vi "GeoData.vi"() -> ()   [LabVIEW 2017] (continued)
GA\tMadison County\tH1\n30530\t13195\tCommerce\tGA\tMadison County\tH1\n30629\t13195\tComer\tGA\tMadison County\tH1\n30624\t13195\tBowman\tGA\tMadison County\tH1\n30601\t13195\tAthens\tGA\tMadison County\tH1\n30646\t13195\tHull\tGA\tMadison County\tH1\n30662\t13195\tRoyston\tGA\tMadison County\tH1\n30647\t13195\tIla\tGA\tMadison County\tH1\n31801\t13197\tBox springs\tGA\tMarion County\tH1\n31805\t13197\tCusseta\tGA\tMarion County\tH1\n31803\t13197\tBuena vista\tGA\tMarion County\tH1\n31058\t13197\tMauk\tGA\tMarion County\tH1\n31824\t13197\tPreston\tGA\tMarion County\tH1\n30241\t13199\tLagrange\tGA\tMeriwether County\tH1\n30251\t13199\tLuthersville\tGA\tMeriwether County\tH1\n30230\t13199\tHogansville\tGA\tMeriwether County\tH1\n30293\t13199\tWoodbury\tGA\tMeriwether County\tH1\n31822\t13199\tPine mountain\tGA\tMeriwether County\tH1\n31816\t13199\tManchester\tGA\tMeriwether County\tH1\n30220\t13199\tGrantville\tGA\tMeriwether County\tH1\n30276\t13199\tSenoia\tGA\tMeriwether County\tH1\n30259\t13199\tMoreland\tGA\tMeriwether County\tH1\n30218\t13199\tGay\tGA\tMeriwether County\tH1\n30222\t13199\tGreenville\tGA\tMeriwether County\tH1\n31830\t13199\tWarm springs\tGA\tMeriwether County\tH1\n39841\t13201\tDamascus\tGA\tMiller County\tH1\n39859\t13201\tIron city\tGA\tMiller County\tH1\n39823\t13201\tBlakely\tGA\tMiller County\tH1\n39845\t13201\tDonalsonville\tGA\tMiller County\tH1\n39837\t13201\tColquitt\tGA\tMiller County\tH1\n31744\t13205\tDoerun\tGA\tMitchell County\tH1\n31779\t13205\tPelham\tGA\tMitchell County\tH1\n31784\t13205\tSale city\tGA\tMitchell County\tH1\n31765\t13205\tMeigs\tGA\tMitchell County\tH1\n31716\t13205\tBaconton\tGA\tMitchell County\tH1\n31705\t13205\tAlbany\tGA\tMitchell County\tH1\n31730\t13205\tCamilla\tGA\tMitchell County\tH1\n31016\t13207\tCulloden\tGA\tMonroe County\tH1\n31097\t13207\tYatesville\tGA\tMonroe County\tH1\n30204\t13207\tBarnesville\tGA\tMonroe County\tH1\n31220\t13207\tMacon\tGA\tMonroe County\tH1\n31029\t13207\tForsyth\tGA\tMonroe County\tH1\n31046\t13207\tJuliette\tGA\tMonroe County\tH1\n31066\t13207\tMusella\tGA\tMonroe County\tH1\n31086\t13207\tSmarr\tGA\tMonroe County\tH1\n30233\t13207\tJackson\tGA\tMonroe County\tH1\n31210\t13207\tMacon\tGA\tMonroe County\tH1\n31004\t13207\tBolingbroke\tGA\tMonroe County\tH1\n30457\t13209\tSoperton\tGA\tMontgomery County\tH1\n30445\t13209\tMount vernon\tGA\tMontgomery County\tH1\n30470\t13209\tTarrytown\tGA\tMontgomery County\tH1\n30410\t13209\tAiley\tGA\tMontgomery County\tH1\n30473\t13209\tUvalda\tGA\tMontgomery County\tH1\n30412\t13209\tAlston\tGA\tMontgomery County\tH1\n30474\t13209\tVidalia\tGA\tMontgomery County\tH1\n30625\t13211\tBuckhead\tGA\tMorgan County\tH1\n30623\t13211\tBostwick\tGA\tMorgan County\tH1\n30055\t13211\tMansfield\tGA\tMorgan County\tH1\n30650\t13211\tMadison\tGA\tMorgan County\tH1\n30025\t13211\tSocial circle\tGA\tMorgan County\tH1\n30663\t13211\tRutledge\tGA\tMorgan County\tH1\n30056\t13211\tNewborn\tGA\tMorgan County\tH1\n30621\t13211\tBishop\tGA\tMorgan County\tH1\n30641\t13211\tGood hope\tGA\tMorgan County\tH1\n30711\t13213\tCrandall\tGA\tMurray County\tH1\n30705\t13213\tChatsworth\tGA\tMurray County\tH1\n30751\t13213\tTennga\tGA\tMurray County\tH1\n30540\t13213\tEllijay\tGA\tMurray County\tH1\n30708\t13213\tCisco\tGA\tMurray County\tH1\n30735\t13213\tResaca\tGA\tMurray County\tH1\n30721\t13213\tDalton\tGA\tMurray County\tH1\n30724\t13213\tEton\tGA\tMurray County\tH1\n31801\t13215\tBox springs\tGA\tMuscogee County\tH6\n31905\t13215\tFort benning\tGA\tMuscogee County\tH6\n31908\t13215\tColumbus\tGA\tMuscogee County\tH6\n31914\t13215\tColumbus\tGA\tMuscogee County\tH6\n31999\t13215\tColumbus\tGA\tMuscogee County\tH6\n31808\t13215\tFortson\tGA\tMuscogee County\tH6\n31804\t13215\tCataula\tGA\tMuscogee County\tH6\n31901\t13215\tColumbus\tGA\tMuscogee County\tH6\n31917\t13215\tColumbus\tGA\tMuscogee County\tH6\n31998\t13215\tColumbus\tGA\tMuscogee County\tH6\n31903\t13215\tColumbus\tGA\tMuscogee County\tH6\n31904\t13215\tColumbus\tGA\tMuscogee County\tH6\n31909\t13215\tColumbus\tGA\tMuscogee County\tH6\n31902\t13215\tColumbus\tGA\tMuscogee County\tH6\n31820\t13215\tMidland\tGA\tMuscogee County\tH6\n31906\t13215\tColumbus\tGA\tMuscogee County\tH6\n31907\t13215\tColumbus\tGA\tMuscogee County\tH6\n31829\t13215\tUpatoi\tGA\tMuscogee County\tH6\n30014\t13217\tCovington\tGA\tNewton County\tH1\n30016\t13217\tCovington\tGA\tNewton County\tH1\n30013\t13217\tConyers\tGA\tNewton County\tH1\n30055\t13217\tMansfield\tGA\tNewton County\tH1\n31064\t13217\tMonticello\tGA\tNewton County\tH1\n30015\t13217\tCovington\tGA\tNewton County\tH1\n30070\t13217\tPorterdale\tGA\tNewton County\tH1\n30025\t13217\tSocial circle\tGA\tNewton County\tH1\n30052\t13217\tLoganville\tGA\tNewton County\tH1\n30094\t13217\tConyers\tGA\tNewton County\tH1\n30054\t13217\tOxford\tGA\tNewton County\tH1\n30056\t13217\tNewborn\tGA\tNewton County\tH1\n30233\t13217\tJackson\tGA\tNewton County\tH1\n30638\t13219\tFarmington\tGA\tOconee County\tH1\n30677\t13219\tWatkinsville\tGA\tOconee County\tH1\n30605\t13219\tAthens\tGA\tOconee County\tH1\n30606\t13219\tAthens\tGA\tOconee County\tH1\n30622\t13219\tBogart\tGA\tOconee County\tH1\n30619\t13219\tArnoldsville\tGA\tOconee County\tH1\n30645\t13219\tHigh shoals\tGA\tOconee County\tH1\n30680\t13219\tWinder\tGA\tOconee County\tH1\n30666\t13219\tStatham\tGA\tOconee County\tH1\n30621\t13219\tBishop\tGA\tOconee County\tH1\n30630\t13221\tCrawford\tGA\tOglethorpe County\tH1\n30627\t13221\tCarlton\tGA\tOglethorpe County\tH1\n30628\t13221\tColbert\tGA\tOglethorpe County\tH1\n30648\t13221\tLexington\tGA\tOglethorpe County\tH1\n30667\t13221\tStephens\tGA\tOglethorpe County\tH1\n30683\t13221\tWinterville\tGA\tOglethorpe County\tH1\n30619\t13221\tArnoldsville\tGA\tOglethorpe County\tH1\n30629\t13221\tComer\tGA\tOglethorpe County\tH1\n30660\t13221\tRayle\tGA\tOglethorpe County\tH1\n30669\t13221\tUnion point\tGA\tOglethorpe County\tH1\n30134\t13223\tDouglasville\tGA\tPaulding County\tH1\n30132\t13223\tDallas\tGA\tPaulding County\tH1\n30157\t13223\tDallas\tGA\tPaulding County\tH1\n30179\t13223\tTemple\tGA\tPaulding County\tH1\n30127\t13223\tPowder springs\tGA\tPaulding County\tH1\n30178\t13223\tTaylorsville\tGA\tPaulding County\tH1\n30101\t13223\tAcworth\tGA\tPaulding County\tH1\n30180\t13223\tVilla rica\tGA\tPaulding County\tH1\n30120\t13223\tCartersville\tGA\tPaulding County\tH1\n30141\t13223\tHiram\tGA\tPaulding County\tH1\n30153\t13223\tRockmart\tGA\tPaulding County\tH1\n31076\t13225\tReynolds\tGA\tPeach County\tH1\n31069\t13225\tPerry\tGA\tPeach County\tH1\n31008\t13225\tByron\tGA\tPeach County\tH1\n31030\t13225\tFort valley\tGA\tPeach County\tH1\n30534\t13227\tDawsonville\tGA\tPickens County\tH1\n30107\t13227\tBall ground\tGA\tPickens County\tH1\n30536\t13227\tEllijay\tGA\tPickens County\tH1\n30139\t13227\tFairmount\tGA\tPickens County\tH1\n30177\t13227\tTate\tGA\tPickens County\tH1\n30540\t13227\tEllijay\tGA\tPickens County\tH1\n30183\t13227\tWaleska\tGA\tPickens County\tH1\n30734\t13227\tRanger\tGA\tPickens County\tH1\n30143\t13227\tJasper\tGA\tPickens County\tH1\n30148\t13227\tMarble hill\tGA\tPickens County\tH1\n30175\t13227\tTalking rock\tGA\tPickens County\tH1\n31551\t13229\tMershon\tGA\tPierce County\tH1\n31557\t13229\tPatterson\tGA\tPierce County\tH1\n31518\t13229\tBristol\tGA\tPierce County\tH1\n31556\t13229\tOfferman\tGA\tPierce County\tH1\n31516\t13229\tBlackshear\tGA\tPierce County\tH1\n31503\t13229\tWaycross\tGA\tPierce County\tH1\n31510\t13229\tAlma\tGA\tPierce County\tH1\n30206\t13231\tConcord\tGA\tPike County\tH1\n30295\t13231\tZebulon\tGA\tPike County\tH1\n30224\t13231\tGriffin\tGA\tPike County\tH1\n30258\t13231\tMolena\tGA\tPike County\tH1\n30292\t13231\tWilliamson\tGA\tPike County\tH1\n30257\t13231\tMilner\tGA\tPike County\tH1\n30285\t13231\tThe rock\tGA\tPike County\tH1\n30256\t13231\tMeansville\tGA\tPike County\tH1\n30124\t13233\tCave spring\tGA\tPolk County\tH1\n30147\t13233\tLindale\tGA\tPolk County\tH1\n30138\t13233\tEsom hill\tGA\tPolk County\tH1\n30178\t13233\tTaylorsville\tGA\tPolk County\tH1\n30125\t13233\tCedartown\tGA\tPolk County\tH1\n30104\t13233\tAragon\tGA\tPolk County\tH1\n30173\t13233\tSilver creek\tGA\tPolk County\tH1\n30113\t13233\tBuchanan\tGA\tPolk County\tH1\n30153\t13233\tRockmart\tGA\tPolk County\tH1\n31036\t13235\tHawkinsville\tGA\tPulaski County\tH1\n31071\t13235\tPineview\tGA\tPulaski County\tH1\n31014\t13235\tCochran\tGA\tPulaski County\tH1\n31091\t13235\tUnadilla\tGA\tPulaski County\tH1\n31023\t13235\tEastman\tGA\tPulaski County\tH1\n30625\t13237\tBuckhead\tGA\tPutnam County\tH1\n31026\t13237\tEatonton\tGA\tPutnam County\tH1\n31024\t13237\tEatonton\tGA\tPutnam County\tH1\n30650\t13237\tMadison\tGA\tPutnam County\tH1\n31061\t13237\tMilledgeville\tGA\tPutnam County\tH1\n39854\t13239\tGeorgetown\tGA\tQuitman County\tH1\n39867\t13239\tMorris\tGA\tQuitman County\tH1\n30568\t13241\tRabun gap\tGA\tRabun County\tH1\n30523\t13241\tClarkesville\tGA\tRabun County\tH1\n30537\t13241\tDillard\tGA\tRabun County\tH1\n30562\t13241\tMountain city\tGA\tRabun County\tH1\n30576\t13241\tTiger\tGA\tRabun County\tH1\n30581\t13241\tWiley\tGA\tRabun County\tH1\n30573\t13241\tTallulah falls\tGA\tRabun County\tH1\n30525\t13241\tClayton\tGA\tRabun County\tH1\n30552\t13241\tLakemont\tGA\tRabun County\tH1\n39840\t13243\tCuthbert\tGA\tRandolph County\tH1\n39866\t13243\tMorgan\tGA\tRandolph County\tH1\n39867\t13243\tMorris\tGA\tRandolph County\tH1\n39846\t13243\tEdison\tGA\tRandolph County\tH1\n39886\t13243\tShellman\tGA\tRandolph County\tH1\n39836\t13243\tColeman\tGA\tRandolph County\tH1\n39851\t13243\tFort gaines\tGA\tRandolph County\tH1\n30912\t13245\tAugusta\tGA\tRichmond County\tH6\n30901\t13245\tAugusta\tGA\tRichmond County\tH6\n30909\t13245\tAugusta\tGA\tRichmond County\tH6\n30815\t13245\tHephzibah\tGA\tRichmond County\tH6\n30906\t13245\tAugusta\tGA\tRichmond County\tH6\n30905\t13245\tAugusta\tGA\tRichmond County\tH6\n30812\t13245\tGracewood\tGA\tRichmond County\tH6\n30805\t13245\tBlythe\tGA\tRichmond County\tH6\n30904\t13245\tAugusta\tGA\tRichmond County\tH6\n30907\t13245\tAugusta\tGA\tRichmond County\tH6\n30903\t13245\tAugusta\tGA\tRichmond County\tH6\n30916\t13245\tAugusta\tGA\tRichmond County\tH6\n30919\t13245\tAugusta\tGA\tRichmond County\tH6\n30914\t13245\tAugusta\tGA\tRichmond County\tH6\n30813\t13245\tGrovetown\tGA\tRichmond County\tH6\n30016\t13247\tCovington\tGA\tRockdale County\tH1\n30039\t13247\tSnellville\tGA\tRockdale County\tH1\n30013\t13247\tConyers\tGA\tRockdale County\tH1\n30012\t13247\tConyers\tGA\tRockdale County\tH1\n30294\t13247\tEllenwood\tGA\tRockdale County\tH1\n30058\t13247\tLithonia\tGA\tRockdale County\tH1\n30052\t13247\tLoganville\tGA\tRockdale County\tH1\n30094\t13247\tConyers\tGA\tRockdale County\tH1\n30252\t13247\tMcdonough\tGA\tRockdale County\tH1\n30281\t13247\tStockbridge\tGA\tRockdale County\tH1\n31711\t13249\tAndersonville\tGA\tSchley County\tH1\n31806\t13249\tEllaville\tGA\tSchley County\tH1\n31081\t13249\tRupert\tGA\tSchley County\tH1\n31068\t13249\tOglethorpe\tGA\tSchley County\tH1\n31719\t13249\tAmericus\tGA\tSchley County\tH1\n31803\t13249\tBuena vista\tGA\tSchley County\tH1\n31058\t13249\tMauk\tGA\tSchley County\tH1\n30424\t13251\tDover\tGA\tScreven County\tH1\n30426\t13251\tGirard\tGA\tScreven County\tH1\n30442\t13251\tMillen\tGA\tScreven County\tH1\n30467\t13251\tSylvania\tGA\tScreven County\tH1\n30455\t13251\tRocky ford\tGA\tScreven County\tH1\n30446\t13251\tNewington\tGA\tScreven County\tH1\n30449\t13251\tOliver\tGA\tScreven County\tH1\n39825\t13253\tBrinson\tGA\tSeminole County\tH1\n39859\t13253\tIron city\tGA\tSeminole County\tH1\n39845\t13253\tDonalsonville\tGA\tSeminole County\tH1\n39861\t13253\tJakin\tGA\tSeminole County\tH1\n30223\t13255\tGriffin\tGA\tSpalding County\tH1\n30266\t13255\tOrchard hill\tGA\tSpalding County\tH1\n30284\t13255\tSunny side\tGA\tSpalding County\tH1\n30224\t13255\tGriffin\tGA\tSpalding County\tH1\n30212\t13255\tExperiment\tGA\tSpalding County\tH1\n30228\t13255\tHampton\tGA\tSpalding County\tH1\n30292\t13255\tWilliamson\tGA\tSpalding County\tH1\n30205\t13255\tBrooks\tGA\tSpalding County\tH1\n30248\t13255\tLocust grove\tGA\tSpalding County\tH1\n30598\t13257\tToccoa falls\tGA\tStephens County\tH1\n30557\t13257\tMartin\tGA\tStephens County\tH1\n30538\t13257\tEastanollee\tGA\tStephens County\tH1\n30577\t13257\tToccoa\tGA\tStephens County\tH1\n39854\t13259\tGeorgetown\tGA\tStewart County\tH1\n31825\t13259\tRichland\tGA\tStewart County\tH1\n31805\t13259\tCusseta\tGA\tStewart County\tH1\n39867\t13259\tMorris\tGA\tStewart County\tH1\n31815\t13259\tLumpkin\tGA\tStewart County\tH1\n31821\t13259\tOmaha\tGA\tStewart County\tH1\n31711\t13261\tAndersonville\tGA\tSumter County\tH1\n31806\t13261\tEllaville\tGA\tSumter County\tH1\n31787\t13261\tSmithville\tGA\tSumter County\tH1\n31735\t13261\tCobb\tGA\tSumter County\tH1\n31719\t13261\tAmericus\tGA\tSumter County\tH1\n31709\t13261\tAmericus\tGA\tSumter County\tH1\n31780\t13261\tPlains\tGA\tSumter County\tH1\n31743\t13261\tDe soto\tGA\tSumter County\tH1\n31764\t13261\tLeslie\tGA\tSumter County\tH1\n31801\t13263\tBox springs\tGA\tTalbot County\tH1\n31827\t13263\tTalbotton\tGA\tTalbot County\tH1\n31816\t13263\tManchester\tGA\tTalbot County\tH1\n31826\t13263\tShiloh\tGA\tTalbot County\tH1\n31836\t13263\tWoodland\tGA\tTalbot County\tH1\n31812\t13263\tJunction city\tGA\tTalbot County\tH1\n31810\t13263\tGeneva\tGA\tTalbot County\tH1\n31831\t13263\tWaverly hall\tGA\tTalbot County\tH1\n30673\t13265\tWashington\tGA\tTaliaferro County\tH1\n30678\t13265\tWhite plains\tGA\tTaliaferro County\tH1\n30664\t13265\tSharon\tGA\tTaliaferro County\tH1\n30631\t13265\tCrawfordville\tGA\tTaliaferro County\tH1\n30660\t13265\tRayle\tGA\tTaliaferro County\tH1\n30669\t13265\tUnion point\tGA\tTaliaferro County\tH1\n30420\t13267\tCobbtown\tGA\tTattnall County\tH1\n30421\t13267\tCollins\tGA\tTattnall County\tH1\n30436\t13267\tLyons\tGA\tTattnall County\tH1\n30453\t13267\tReidsville\tGA\tTattnall County\tH1\n30499\t13267\tReidsville\tGA\tTattnall County\tH1\n30417\t13267\tClaxton\tGA\tTattnall County\tH1\n30427\t13267\tGlennville\tGA\tTattnall County\tH1\n30438\t13267\tManassas\tGA\tTattnall County\tH1\n31076\t13269\tReynolds\tGA\tTaylor County\tH1\n31081\t13269\tRupert\tGA\tTaylor County\tH1\n31068\t13269\tOglethorpe\tGA\tTaylor County\tH1\n31041\t13269\tIdeal\tGA\tTaylor County\tH1\n31006\t13269\tButler\tGA\tTaylor County\tH1\n31058\t13269\tMauk\tGA\tTaylor County\tH1\n31812\t13269\tJunction city\tGA\tTaylor County\tH1\n31039\t13269\tHoward\tGA\tTaylor County\tH1\n31037\t13271\tMc rae helena\tGA\tTelfair County\tH1\n31055\t13271\tMc rae helena\tGA\tTelfair County\tH1\n31060\t13271\tMilan\tGA\tTelfair County\tH1\n31549\t13271\tLumber city\tGA\tTelfair County\tH1\n31083\t13271\tScotland\tGA\tTelfair County\tH1\n31077\t13271\tRhine\tGA\tTelfair County\tH1\n31544\t13271\tJacksonville\tGA\tTelfair County\tH1\n31721\t13273\tAlbany\tGA\tTerrell County\tH1\n39842\t13273\tDawson\tGA\tTerrell County\tH1\n39862\t13273\tLeary\tGA\tTerrell County\tH1\n39826\t13273\tBronwood\tGA\tTerrell County\tH1\n39886\t13273\tShellman\tGA\tTerrell County\tH1\n39877\t13273\tParrott\tGA\tTerrell County\tH1\n39885\t13273\tSasser\tGA\tTerrell County\tH1\n31738\t13275\tCoolidge\tGA\tThomas County\tH1\n31720\t13275\tBarwick\tGA\tThomas County\tH1\n31779\t13275\tPelham\tGA\tThomas County\tH1\n31778\t13275\tPavo\tGA\tThomas County\tH1\n31773\t13275\tOchlocknee\tGA\tThomas County\tH1\n31792\t13275\tThomasville\tGA\tThomas County\tH1\n31757\t13275\tThomasville\tGA\tThomas County\tH1\n31765\t13275\tMeigs\tGA\tThomas County\tH1\n39828\t13275\tCairo\tGA\tThomas County\tH1\n31799\t13275\tThomasville\tGA\tThomas County\tH1\n31626\t13275\tBoston\tGA\tThomas County\tH1\n31733\t13277\tChula\tGA\tTift County\tH1\n31775\t13277\tOmega\tGA\tTift County\tH1\n31793\t13277\tTifton\tGA\tTift County\tH1\n31714\t13277\tAshburn\tGA\tTift County\tH1\n31790\t13277\tSycamore\tGA\tTift County\tH1\n31637\t13277\tLenox\tGA\tTift County\tH1\n31795\t13277\tTy ty\tGA\tTift County\tH1\n31727\t13277\tBrookfield\tGA\tTift County\tH1\n31749\t13277\tEnigma\tGA\tTift County\tH1\n31794\t13277\tTifton\tGA\tTift County\tH1\n30436\t13279\tLyons\tGA\tToombs County\tH1\n30453\t13279\tReidsville\tGA\tToombs County\tH1\n30473\t13279\tUvalda\tGA\tToombs County\tH1\n30474\t13279\tVidalia\tGA\tToombs County\tH1\n30582\t13281\tYoung harris\tGA\tTowns County\tH1\n30525\t13281\tClayton\tGA\tTowns County\tH1\n30546\t13281\tHiawassee\tGA\tTowns County\tH1\n30457\t13283\tSoperton\tGA\tTreutlen County\tH1\n31002\t13283\tAdrian\tGA\tTreutlen County\tH1\n30470\t13283\tTarrytown\tGA\tTreutlen County\tH1\n30436\t13283\tLyons\tGA\tTreutlen County\tH1\n30474\t13283\tVidalia\tGA\tTreutlen County\tH1\n30241\t13285\tLagrange\tGA\tTroup County\tH1\n30217\t13285\tFranklin\tGA\tTroup County\tH1\n30261\t13285\tLagrange\tGA\tTroup County\tH1\n30230\t13285\tHogansville\tGA\tTroup County\tH1\n31822\t13285\tPine mountain\tGA\tTroup County\tH1\n30220\t13285\tGrantville\tGA\tTroup County\tH1\n30240\t13285\tLagrange\tGA\tTroup County\tH1\n31833\t13285\tWest point\tGA\tTroup County\tH1\n31714\t13287\tAshburn\tGA\tTurner County\tH1\n31790\t13287\tSycamore\tGA\tTurner County\tH1\n31789\t13287\tSumner\tGA\tTurner County\tH1\n31712\t13287\tArabi\tGA\tTurner County\tH1\n31783\t13287\tRebecca\tGA\tTurner County\tH1\n31031\t13289\tGordon\tGA\tTwiggs County\tH1\n31044\t13289\tJeffersonville\tGA\tTwiggs County\tH1\n31014\t13289\tCochran\tGA\tTwiggs County\tH1\n31017\t13289\tDanville\tGA\tTwiggs County\tH1\n31217\t13289\tMacon\tGA\tTwiggs County\tH1\n31020\t13289\tDry branch\tGA\tTwiggs County\tH1\n30514\t13291\tBlairsville\tGA\tUnion County\tH1\n30572\t13291\tSuches\tGA\tUnion County\tH1\n30560\t13291\tMorganton\tGA\tUnion County\tH1\n30512\t13291\tBlairsville\tGA\tUnion County\tH1\n30582\t13291\tYoung harris\tGA\tUnion County\tH1\n30513\t13291\tBlue ridge\tGA\tUnion County\tH1\n30546\t13291\tHiawassee\tGA\tUnion County\tH1\n31016\t13293\tCulloden\tGA\tUpson County\tH1\n31097\t13293\tYatesville\tGA\tUpson County\tH1\n30204\t13293\tBarnesville\tGA\tUpson County\tH1\n30258\t13293\tMolena\tGA\tUpson County\tH1\n30285\t13293\tThe rock\tGA\tUpson County\tH1\n30286\t13293\tThomaston\tGA\tUpson County\tH1\n30256\t13293\tMeansville\tGA\tUpson County\tH1\n30752\t13295\tTrenton\tGA\tWalker County\tH1\n30725\t13295\tFlintstone\tGA\tWalker County\tH1\n30707\t13295\tChickamauga\tGA\tWalker County\tH1\n30746\t13295\tSugar valley\tGA\tWalker County\tH1\n30741\t13295\tRossville\tGA\tWalker County\tH1\n30738\t13295\tRising fawn\tGA\tWalker County\tH1\n30736\t13295\tRinggold\tGA\tWalker County\tH1\n30742\t13295\tFort oglethorpe\tGA\tWalker County\tH1\n30728\t13295\tLa fayette\tGA\tWalker County\tH1\n30750\t13295\tLookout mountain\tGA\tWalker County\tH1\n30739\t13295\tRock spring\tGA\tWalker County\tH1\n30731\t13295\tMenlo\tGA\tWalker County\tH1\n30753\t13295\tTrion\tGA\tWalker County\tH1\n30747\t13295\tSummerville\tGA\tWalker County\tH1\n30740\t13295\tRocky face\tGA\tWalker County\tH1\n30014\t13297\tCovington\tGA\tWalton County\tH1\n30620\t13297\tBethlehem\tGA\tWalton County\tH1\n30018\t13297\tJersey\tGA\tWalton County\tH1\n30012\t13297\tConyers\tGA\tWalton County\tH1\n30650\t13297\tMadison\tGA\tWalton County\tH1\n30656\t13297\tMonroe\tGA\tWalton County\tH1\n30025\t13297\tSocial circle\tGA\tWalton County\tH1\n30052\t13297\tLoganville\tGA\tWalton County\tH1\n30655\t13297\tMonroe\tGA\tWalton County\tH1\n30663\t13297\tRutledge\tGA\tWalton County\tH1\n30054\t13297\tOxford\tGA\tWalton County\tH1\n30641\t13297\tGood hope\tGA\tWalton County\tH1\n30019\t13297\tDacula\tGA\tWalton County\tH1\n31552\t13299\tMillwood\tGA\tWare County\tH1\n31502\t13299\tWaycross\tGA\tWare County\tH1\n31624\t13299\tAxson\tGA\tWare County\tH1\n31631\t13299\tFargo\tGA\tWare County\tH1\n31564\t13299\tWaresboro\tGA\tWare County\tH1\n31554\t13299\tNicholls\tGA\tWare County\tH1\n31503\t13299\tWaycross\tGA\tWare County\tH1\n31501\t13299\tWaycross\tGA\tWare County\tH1\n31550\t13299\tManor\tGA\tWare County\tH1\n31510\t13299\tAlma\tGA\tWare County\tH1\n30824\t13301\tThomson\tGA\tWarren County\tH1\n30810\t13301\tGibson\tGA\tWarren County\tH1\n31045\t13301\tJewell\tGA\tWarren County\tH1\n30821\t13301\tNorwood\tGA\tWarren County\tH1\n30828\t13301\tWarrenton\tGA\tWarren County\tH1\n30823\t13301\tStapleton\tGA\tWarren County\tH1\n30820\t13301\tMitchell\tGA\tWarren County\tH1\n30807\t13301\tCamak\tGA\tWarren County\tH1\n30819\t13301\tMesena\tGA\tWarren County\tH1\n31096\t13303\tWrightsville\tGA\tWashington County\tH1\n31094\t13303\tWarthen\tGA\tWashington County\tH1\n31035\t13303\tHarrison\tGA\tWashington County\tH1\n31089\t13303\tTennille\tGA\tWashington County\tH1\n31067\t13303\tOconee\tGA\tWashington County\tH1\n31082\t13303\tSandersville\tGA\tWashington County\tH1\n31018\t13303\tDavisboro\tGA\tWashington County\tH1\n30413\t13303\tBartow\tGA\tWashington County\tH1\n30820\t13303\tMitchell\tGA\tWashington County\tH1\n31087\t13303\tSparta\tGA\tWashington County\tH1\n31543\t13305\tHortense\tGA\tWayne County\tH1\n31518\t13305\tBristol\tGA\tWayne County\tH1\n31560\t13305\tScreven\tGA\tWayne County\tH1\n31599\t13305\tJesup\tGA\tWayne County\tH1\n31546\t13305\tJesup\tGA\tWayne County\tH1\n31545\t13305\tJesup\tGA\tWayne County\tH1\n31555\t13305\tOdum\tGA\tWayne County\tH1\n31598\t13305\tJesup\tGA\tWayne County\tH1\n31825\t13307\tRichland\tGA\tWebster County\tH1\n31832\t13307\tWeston\tGA\tWebster County\tH1\n31780\t13307\tPlains\tGA\tWebster County\tH1\n31803\t13307\tBuena vista\tGA\tWebster County\tH1\n31824\t13307\tPreston\tGA\tWebster County\tH1\n39877\t13307\tParrott\tGA\tWebster County\tH1\n30411\t13309\tAlamo\tGA\tWheeler County\tH1\n31037\t13309\tMc rae helena\tGA\tWheeler County\tH1\n31549\t13309\tLumber city\tGA\tWheeler County\tH1\n30428\t13309\tGlenwood\tGA\tWheeler County\tH1\n30527\t13311\tClermont\tGA\tWhite County\tH1\n30564\t13311\tMurrayville\tGA\tWhite County\tH1\n30523\t13311\tClarkesville\tGA\tWhite County\tH1\n30533\t13311\tDahlonega\tGA\tWhite County\tH1\n30545\t13311\tHelen\tGA\tWhite County\tH1\n30571\t13311\tSautee nacoochee\tGA\tWhite County\tH1\n30528\t13311\tCleveland\tGA\tWhite County\tH1\n30554\t13311\tLula\tGA\tWhite County\tH1\n30722\t13313\tDalton\tGA\tWhitfield County\tH1\n30720\t13313\tDalton\tGA\tWhitfield County\tH1\n30719\t13313\tDalton\tGA\tWhitfield County\tH1\n30736\t13313\tRinggold\tGA\tWhitfield County\tH1\n30710\t13313\tCohutta\tGA\tWhitfield County\tH1\n30755\t13313\tTunnel hill\tGA\tWhitfield County\tH1\n30756\t13313\tVarnell\tGA\tWhitfield County\tH1\n30735\t13313\tResaca\tGA\tWhitfield County\tH1\n30721\t13313\tDalton\tGA\tWhitfield County\tH1\n30740\t13313\tRocky face\tGA\tWhitfield County\tH1\n31072\t13315\tPitts\tGA\tWilcox County\tH1\n31001\t13315\tAbbeville\tGA\tWilcox County\tH1\n31092\t13315\tVienna\tGA\tWilcox County\tH1\n31015\t13315\tCordele\tGA\tWilcox County\tH1\n31071\t13315\tPineview\tGA\tWilcox County\tH1\n31079\t13315\tRochelle\tGA\tWilcox County\tH1\n31750\t13315\tFitzgerald\tGA\tWilcox County\tH1\n30817\t13317\tLincolnton\tGA\tWilkes County\tH1\n30668\t13317\tTignall\tGA\tWilkes County\tH1\n30673\t13317\tWashington\tGA\tWilkes County\tH1\n30631\t13317\tCrawfordville\tGA\tWilkes County\tH1\n30660\t13317\tRayle\tGA\tWilkes County\tH1\n31021\t13319\tDublin\tGA\tWilkinson County\tH1\n31031\t13319\tGordon\tGA\tWilkinson County\tH1\n31044\t13319\tJeffersonville\tGA\tWilkinson County\tH1\n31090\t13319\tToomsboro\tGA\tWilkinson County\tH1\n31017\t13319\tDanville\tGA\tWilkinson County\tH1\n31061\t13319\tMilledgeville\tGA\tWilkinson County\tH1\n31054\t13319\tMc intyre\tGA\tWilkinson County\tH1\n31003\t13319\tAllentown\tGA\tWilkinson County\tH1\n31042\t13319\tIrwinton\tGA\tWilkinson County\tH1\n31065\t13319\tMontrose\tGA\tWilkinson County\tH1\n31791\t13321\tSylvester\tGA\tWorth County\tH1\n31744\t13321\tDoerun\tGA\tWorth County\tH1\n31775\t13321\tOmega\tGA\tWorth County\tH1\n31772\t13321\tOakfield\tGA\tWorth County\tH1\n31714\t13321\tAshburn\tGA\tWorth County\tH1\n31768\t13321\tMoultrie\tGA\tWorth County\tH1\n31789\t13321\tSumner\tGA\tWorth County\tH1\n31796\t13321\tWarwick\tGA\tWorth County\tH1\n31712\t13321\tArabi\tGA\tWorth County\tH1\n31771\t13321\tNorman park\tGA\tWorth County\tH1\n31795\t13321\tTy ty\tGA\tWorth County\tH1\n31705\t13321\tAlbany\tGA\tWorth County\tH1\n31781\t13321\tPoulan\tGA\tWorth County\tH1\n96740\t15001\tKailua kona\tHI\tHawaii County\tH1\n96783\t15001\tPepeekeo\tHI\tHawaii County\tH1\n96739\t15001\tKeauhou\tHI\tHawaii County\tH1\n96764\t15001\tLaupahoehoe\tHI\tHawaii County\tH1\n96725\t15001\tHolualoa\tHI\tHawaii County\tH1\n96718\t15001\tHawaii national park\tHI\tHawaii County\tH1\n96710\t15001\tHakalau\tHI\tHawaii County\tH1\n96773\t15001\tNinole\tHI\tHawaii County\tH1\n96743\t15001\tKamuela\tHI\tHawaii County\tH1\n96760\t15001\tKurtistown\tHI\tHawaii County\tH1\n96781\t15001\tPapaikou\tHI\tHawaii County\tH1\n96738\t15001\tWaikoloa\tHI\tHawaii County\tH1\n96771\t15001\tMountain view\tHI\tHawaii County\tH1\n96750\t15001\tKealakekua\tHI\tHawaii County\tH1\n96728\t15001\tHonomu\tHI\tHawaii County\tH1\n96727\t15001\tHonokaa\tHI\tHawaii County\tH1\n96721\t15001\tHilo\tHI\tHawaii County\tH1\n96755\t15001\tKapaau\tHI\tHawaii County\tH1\n96777\t15001\tPahala\tHI\tHawaii County\tH1\n96774\t15001\tOokala\tHI\tHawaii County\tH1\n96776\t15001\tPaauilo\tHI\tHawaii County\tH1\n96780\t15001\tPapaaloa\tHI\tHawaii County\tH1\n96745\t15001\tKailua kona\tHI\tHawaii County\tH1\n96772\t15001\tNaalehu\tHI\tHawaii County\tH1\n96726\t15001\tHonaunau\tHI\tHawaii County\tH1\n96704\t15001\tCaptain cook\tHI\tHawaii County\tH1\n96720\t15001\tHilo\tHI\tHawaii County\tH1\n96749\t15001\tKeaau\tHI\tHawaii County\tH1\n96778\t15001\tPahoa\tHI\tHawaii County\tH1\n96719\t15001\tHawi\tHI\tHawaii County\tH1\n96737\t15001\tOcean view\tHI\tHawaii County\tH1\n96785\t15001\tVolcano\tHI\tHawaii County\tH1\n96792\t15003\tWaianae\tHI\tHonolulu County\tH1\n96854\t15003\tWheeler army airfield\tHI\tHonolulu County\tH1\n96709\t15003\tKapolei\tHI\tHonolulu County\tH1\n96812\t15003\tHonolulu\tHI\tHonolulu County\tH1\n96730\t15003\tKaaawa\tHI\tHonolulu County\tH1\n96857\t15003\tSchofield barracks\tHI\tHonolulu County\tH1\n96701\t15003\tAiea\tHI\tHonolulu County\tH1\n96795\t15003\tWaimanalo\tHI\tHonolulu County\tH1\n96822\t15003\tHonolulu\tHI\tHonolulu County\tH1\n96860\t15003\tJbphh\tHI\tHonolulu County\tH1\n96823\t15003\tHonolulu\tHI\tHonolulu County\tH1\n96802\t15003\tHonolulu\tHI\tHonolulu County\tH1\n96804\t15003\tHonolulu\tHI\tHonolulu County\tH1\n96806\t15003\tHonolulu\tHI\tHonolulu County\tH1\n96706\t15003\tEwa beach\tHI\tHonolulu County\tH1\n96817\t15003\tHonolulu\tHI\tHonolulu County\tH1\n96839\t15003\tHonolulu\tHI\tHonolulu County\tH1\n96712\t15003\tHaleiwa\tHI\tHonolulu County\tH1\n96820\t15003\tHonolulu\tHI\tHonolulu County\tH1\n96824\t15003\tHonolulu\tHI\tHonolulu County\tH1\n96828\t15003\tHonolulu\tHI\tHonolulu County\tH1\n96848\t15003\tHonolulu\tHI\tHonolulu County\tH1\n96858\t15003\tFort shafter\tHI\tHonolulu County\tH1\n96801\t15003\tHonolulu\tHI\tHonolulu County\tH1\n96811\t15003\tHonolulu\tHI\tHonolulu County\tH1\n96859\t15003\tTripler army medical center\tHI\tHonolulu County\tH1\n96797\t15003\tWaipahu\tHI\tHonolulu County\tH1\n96782\t15003\tPearl city\tHI\tHonolulu County\tH1\n96825\t15003\tHonolulu\tHI\tHonolulu County\tH1\n96853\t15003\tJbphh\tHI\tHonolulu County\tH1\n96808\t15003\tHonolulu\tHI\tHonolulu County\tH1\n96810\t15003\tHonolulu\tHI\tHonolulu County\tH1\n96861\t15003\tCamp h m smith\tHI\tHonolulu County\tH1\n96898\t15003\tWake island\tHI\tHonolulu County\tH1\n96734\t15003\tKailua\tHI\tHonolulu County\tH1\n96826\t15003\tHonolulu\tHI\tHonolulu County\tH1\n96863\t15003\tMcbh kaneohe bay\tHI\tHonolulu County\tH1\n96805\t15003\tHonolulu\tHI\tHonolulu County\tH1\n96707\t15003\tKapolei\tHI\tHonolulu County\tH1\n96819\t15003\tHonolulu\tHI\tHonolulu County\tH1\n96821\t15003\tHonolulu\tHI\tHonolulu County\tH1\n96717\t15003\tHauula\tHI\tHonolulu County\tH1\n96807\t15003\tHonolulu\tHI\tHonolulu County\tH1\n96850\t15003\tHonolulu\tHI\tHonolulu County\tH1\n96759\t15003\tKunia\tHI\tHonolulu County\tH1\n96731\t15003\tKahuku\tHI\tHonolulu County\tH1\n96814\t15003\tHonolulu\tHI\tHonolulu County\tH1\n96786\t15003\tWahiawa\tHI\tHonolulu County\tH1\n96813\t15003\tHonolulu\tHI\tHonolulu County\tH1\n96830\t15003\tHonolulu\tHI\tHonolulu County\tH1\n96836\t15003\tHonolulu\tHI\tHonolulu County\tH1\n96837\t15003\tHonolulu\tHI\tHonolulu County\tH1\n96803\t15003\tHonolulu\tHI\tHonolulu County\tH1\n96809\t15003\tHonolulu\tHI\tHonolulu County\tH1\n96744\t15003\tKaneohe\tHI\tHonolulu County\tH1\n96791\t15003\tWaialua\tHI\tHonolulu County\tH1\n96816\t15003\tHonolulu\tHI\tHonolulu County\tH1\n96789\t15003\tMililani\tHI\tHonolulu County\tH1\n96815\t15003\tHonolulu\tHI\tHonolulu County\tH1\n96818\t15003\tHonolulu\tHI\tHonolulu County\tH1\n96762\t15003\tLaie\tHI\tHonolulu County\tH1\n96742\t15005\tKalaupapa\tHI\tKalawao County\tH4\n96754\t15007\tKilauea\tHI\tKauai County\tH1\n96703\t15007\tAnahola\tHI\tKauai County\tH1\n96722\t15007\tPrinceville\tHI\tKauai County\tH1\n96716\t15007\tHanapepe\tHI\tKauai County\tH1\n96747\t15007\tKaumakani\tHI\tKauai County\tH1\n96746\t15007\tKapaa\tHI\tKauai County\tH1\n96751\t15007\tKealia\tHI\tKauai County\tH1\n96766\t15007\tLihue\tHI\tKauai County\tH1\n96715\t15007\tHanamaulu\tHI\tKauai County\tH1\n96705\t15007\tEleele\tHI\tKauai County\tH1\n96765\t15007\tLawai\tHI\tKauai County\tH1\n96741\t15007\tKalaheo\tHI\tKauai County\tH1\n96756\t15007\tKoloa\tHI\tKauai County\tH1\n96714\t15007\tHanalei\tHI\tKauai County\tH1\n96769\t15007\tMakaweli\tHI\tKauai County\tH1\n96796\t15007\tWaimea\tHI\tKauai County\tH1\n96752\t15007\tKekaha\tHI\tKauai County\tH1\n96748\t15009\tKaunakakai\tHI\tMaui County\tH1\n96732\t15009\tKahului\tHI\tMaui County\tH1\n96729\t15009\tHoolehua\tHI\tMaui County\tH1\n96763\t15009\tLanai city\tHI\tMaui County\tH1\n96770\t15009\tMaunaloa\tHI\tMaui County\tH1\n96733\t15009\tKahului\tHI\tMaui County\tH1\n96793\t15009\tWailuku\tHI\tMaui County\tH1\n96768\t15009\tMakawao\tHI\tMaui County\tH1\n96788\t15009\tPukalani\tHI\tMaui County\tH1\n96713\t15009\tHana\tHI\tMaui County\tH1\n96708\t15009\tHaiku\tHI\tMaui County\tH1\n96753\t15009\tKihei\tHI\tMaui County\tH1\n96767\t15009\tLahaina\tHI\tMaui County\tH1\n96779\t15009\tPaia\tHI\tMaui County\tH1\n96761\t15009\tLahaina\tHI\tMaui County\tH1\n96757\t15009\tKualapuu\tHI\tMaui County\tH1\n96784\t15009\tPuunene\tHI\tMaui County\tH1\n96790\t15009\tKula\tHI\tMaui County\tH1\n83642\t16001\tMeridian\tID\tAda County\tH1\n83705\t16001\tBoise\tID\tAda County\tH1\n83707\t16001\tBoise\tID\tAda County\tH1\n83729\t16001\tBoise\tID\tAda County\tH1\n83641\t16001\tMelba\tID\tAda County\tH1\n83669\t16001\tStar\tID\tAda County\tH1\n83704\t16001\tBoise\tID\tAda County\tH1\n83702\t16001\tBoise\tID\tAda County\tH1\n83687\t16001\tNampa\tID\tAda County\tH1\n83724\t16001\tBoise\tID\tAda County\tH1\n83680\t16001\tMeridian\tID\tAda County\tH1\n83717\t16001\tBoise\tID\tAda County\tH1\n83720\t16001\tBoise\tID\tAda County\tH1\n83708\t16001\tBoise\tID\tAda County\tH1\n83712\t16001\tBoise\tID\tAda County\tH1\n83713\t16001\tBoise\tID\tAda County\tH1\n83715\t16001\tBoise\tID\tAda County\tH1\n83728\t16001\tBoise\tID\tAda County\tH1\n83719\t16001\tBoise\tID\tAda County\tH1\n83634\t16001\tKuna\tID\tAda County\tH1\n83646\t16001\tMeridian\tID\tAda County\tH1\n83701\t16001\tBoise\tID\tAda County\tH1\n83709\t16001\tBoise\tID\tAda County\tH1\n83703\t16001\tBoise\tID\tAda County\tH1\n83714\t16001\tGarden city\tID\tAda County\tH1\n83711\t16001\tBoise\tID\tAda County\tH1\n83616\t16001\tEagle\tID\tAda County\tH1\n83706\t16001\tBoise\tID\tAda County\tH1\n83716\t16001\tBoise\tID\tAda County\tH1\n83725\t16001\tBoise\tID\tAda County\tH1\n83735\t16001\tBoise\tID\tAda County\tH1\n83638\t16003\tMccall\tID\tAdams County\tH1\n83612\t16003\tCouncil\tID\tAdams County\tH1\n83632\t16003\tIndian valley\tID\tAdams County\tH1\n83547\t16003\tPollock\tID\tAdams County\tH1\n83643\t16003\tMesa\tID\tAdams County\tH1\n83654\t16003\tNew meadows\tID\tAdams County\tH1\n83205\t16005\tPocatello\tID\tBannock County\tH1\n83214\t16005\tArimo\tID\tBannock County\tH1\n83234\t16005\tDowney\tID\tBannock County\tH1\n83202\t16005\tPocatello\tID\tBannock County\tH1\n83204\t16005\tPocatello\tID\tBannock County\tH1\n83245\t16005\tInkom\tID\tBannock County\tH1\n83281\t16005\tSwanlake\tID\tBannock County\tH1\n83201\t16005\tPocatello\tID\tBannock County\tH1\n83246\t16005\tLava hot springs\tID\tBannock County\tH1\n83209\t16005\tPocatello\tID\tBannock County\tH1\n83250\t16005\tMccammon\tID\tBannock County\tH1\n83206\t16005\tPocatello\tID\tBannock County\tH1\n83238\t16007\tGeneva\tID\tBear Lake County\tH1\n83239\t16007\tGeorgetown\tID\tBear Lake County\tH1\n83254\t16007\tMontpelier\tID\tBear Lake County\tH1\n83287\t16007\tFish haven\tID\tBear Lake County\tH1\n83223\t16007\tBloomington\tID\tBear Lake County\tH1\n83233\t16007\tDingle\tID\tBear Lake County\tH1\n83261\t16007\tParis\tID\tBear Lake County\tH1\n83272\t16007\tSaint charles\tID\tBear Lake County\tH1\n83220\t16007\tBern\tID\tBear Lake County\tH1\n83276\t16007\tSoda springs\tID\tBear Lake County\tH1\n83830\t16009\tFernwood\tID\tBenewah County\tH1\n83870\t16009\tTensed\tID\tBenewah County\tH1\n83876\t16009\tWorley\tID\tBenewah County\tH1\n83866\t16009\tSanta\tID\tBenewah County\tH1\n83861\t16009\tSaint maries\tID\tBenewah County\tH1\n83824\t16009\tDesmet\tID\tBenewah County\tH1\n83851\t16009\tPlummer\tID\tBenewah County\tH1\n83833\t16009\tHarrison\tID\tBenewah County\tH1\n83236\t16011\tFirth\tID\tBingham County\tH1\n83202\t16011\tPocatello\tID\tBingham County\tH1\n83274\t16011\tShelley\tID\tBingham County\tH1\n83211\t16011\tAmerican falls\tID\tBingham County\tH1\n83215\t16011\tAtomic city\tID\tBingham County\tH1\n83203\t16011\tFort hall\tID\tBingham County\tH1\n83404\t16011\tIdaho falls\tID\tBingham County\tH1\n83210\t16011\tAberdeen\tID\tBingham County\tH1\n83402\t16011\tIdaho falls\tID\tBingham County\tH1\n83277\t16011\tSpringfield\tID\tBingham County\tH1\n83218\t16011\tBasalt\tID\tBingham County\tH1\n83221\t16011\tBlackfoot\tID\tBingham County\tH1\n83256\t16011\tMoreland\tID\tBingham County\tH1\n83262\t16011\tPingree\tID\tBingham County\tH1\n83354\t16013\tSun valley\tID\tBlaine County\tH1\n83340\t16013\tKetchum\tID\tBlaine County\tH1\n83333\t16013\tHailey\tID\tBlaine County\tH1\n83313\t16013\tBellevue\tID\tBlaine County\tH1\n83348\t16013\tPicabo\tID\tBlaine County\tH1\n83353\t16013\tSun valley\tID\tBlaine County\tH1\n83320\t16013\tCarey\tID\tBlaine County\tH1\n83637\t16015\tLowman\tID\tBoise County\tH1\n83629\t16015\tHorseshoe bend\tID\tBoise County\tH1\n83702\t16015\tBoise\tID\tBoise County\tH1\n83631\t16015\tIdaho city\tID\tBoise County\tH1\n83622\t16015\tGarden valley\tID\tBoise County\tH1\n83666\t16015\tPlacerville\tID\tBoise County\tH1\n83670\t16015\tSweet\tID\tBoise County\tH1\n83716\t16015\tBoise\tID\tBoise County\tH1\n83602\t16015\tBanks\tID\tBoise County\tH1\n83822\t16017\tOldtown\tID\tBonner County\tH1\n83804\t16017\tBlanchard\tID\tBonner County\tH1\n83813\t16017\tCocolalla\tID\tBonner County\tH1\n83860\t16017\tSagle\tID\tBonner County\tH1\n83864\t16017\tSandpoint\tID\tBonner County\tH1\n83856\t16017\tPriest river\tID\tBonner County\tH1\n83825\t16017\tDover\tID\tBonner County\tH1\n83811\t16017\tClark fork\tID\tBonner County\tH1\n83803\t16017\tBayview\tID\tBonner County\tH1\n83852\t16017\tPonderay\tID\tBonner County\tH1\n83836\t16017\tHope\tID\tBonner County\tH1\n83821\t16017\tCoolin\tID\tBonner County\tH1\n83848\t16017\tNordman\tID\tBonner County\tH1\n83869\t16017\tSpirit lake\tID\tBonner County\tH1\n83801\t16017\tAthol\tID\tBonner County\tH1\n83840\t16017\tKootenai\tID\tBonner County\tH1\n83865\t16017\tColburn\tID\tBonner County\tH1\n83809\t16017\tCareywood\tID\tBonner County\tH1\n83841\t16017\tLaclede\tID\tBonner County\tH1\n83442\t16019\tRigby\tID\tBonneville County\tH1\n83443\t16019\tRirie\tID\tBonneville County\tH1\n83454\t16019\tUcon\tID\tBonneville County\tH1\n83274\t16019\tShelley\tID\tBonneville County\tH1\n83406\t16019\tIdaho falls\tID\tBonneville County\tH1\n83404\t16019\tIdaho falls\tID\tBonneville County\tH1\n83444\t16019\tRoberts\tID\tBonneville County\tH1\n83403\t16019\tIdaho falls\tID\tBonneville County\tH1\n83428\t16019\tIrwin\tID\tBonneville County\tH1\n83285\t16019\tWayan\tID\tBonneville County\tH1\n83401\t16019\tIdaho falls\tID\tBonneville County\tH1\n83402\t16019\tIdaho falls\tID\tBonneville County\tH1\n83427\t16019\tIona\tID\tBonneville County\tH1\n83405\t16019\tIdaho falls\tID\tBonneville County\tH1\n83449\t16019\tSwan valley\tID\tBonneville County\tH1\n83805\t16021\tBonners ferry\tID\tBoundary County\tH1\n83826\t16021\tEastport\tID\tBoundary County\tH1\n83845\t16021\tMoyie springs\tID\tBoundary County\tH1\n83847\t16021\tNaples\tID\tBoundary County\tH1\n83853\t16021\tPorthill\tID\tBoundary County\tH1\n83244\t16023\tHowe\tID\tButte County\tH1\n83255\t16023\tMoore\tID\tButte County\tH1\n83213\t16023\tArco\tID\tButte County\tH1\n83322\t16025\tCorral\tID\tCamas County\tH1\n83327\t16025\tFairfield\tID\tCamas County\tH1\n83686\t16027\tNampa\tID\tCanyon County\tH1\n83651\t16027\tNampa\tID\tCanyon County\tH1\n83641\t16027\tMelba\tID\tCanyon County\tH1\n83669\t16027\tStar\tID\tCanyon County\tH1\n83660\t16027\tParma\tID\tCanyon County\tH1\n83676\t16027\tWilder\tID\tCanyon County\tH1\n83656\t16027\tNotus\tID\tCanyon County\tH1\n83687\t16027\tNampa\tID\tCanyon County\tH1\n83644\t16027\tMiddleton\tID\tCanyon County\tH1\n83634\t16027\tKuna\tID\tCanyon County\tH1\n83607\t16027\tCaldwell\tID\tCanyon County\tH1\n83605\t16027\tCaldwell\tID\tCanyon County\tH1\n83630\t16027\tHuston\tID\tCanyon County\tH1\n83626\t16027\tGreenleaf\tID\tCanyon County\tH1\n83653\t16027\tNampa\tID\tCanyon County\tH1\n83606\t16027\tCaldwell\tID\tCanyon County\tH1\n83217\t16029\tBancroft\tID\tCaribou County\tH1\n83285\t16029\tWayan\tID\tCaribou County\tH1\n83241\t16029\tGrace\tID\tCaribou County\tH1\n83276\t16029\tSoda springs\tID\tCaribou County\tH1\n83318\t16031\tBurley\tID\tCassia County\tH1\n83211\t16031\tAmerican falls\tID\tCassia County\tH1\n83346\t16031\tOakley\tID\tCassia County\tH1\n83323\t16031\tDeclo\tID\tCassia County\tH1\n83342\t16031\tMalta\tID\tCassia County\tH1\n83350\t16031\tRupert\tID\tCassia County\tH1\n83344\t16031\tMurtaugh\tID\tCassia County\tH1\n83311\t16031\tAlbion\tID\tCassia County\tH1\n83312\t16031\tAlmo\tID\tCassia County\tH1\n83423\t16033\tDubois\tID\tClark County\tH1\n83446\t16033\tSpencer\tID\tClark County\tH1\n83435\t16033\tMonteview\tID\tClark County\tH1\n83544\t16035\tOrofino\tID\tClearwater County\tH1\n83546\t16035\tPierce\tID\tClearwater County\tH1\n83553\t16035\tWeippe\tID\tClearwater County\tH1\n83520\t16035\tAhsahka\tID\tClearwater County\tH1\n83545\t16035\tPeck\tID\tClearwater County\tH1\n83827\t16035\tElk river\tID\tClearwater County\tH1\n83541\t16035\tLenore\tID\tClearwater County\tH1\n83537\t16035\tKendrick\tID\tClearwater County\tH1\n83253\t16037\tMay\tID\tCuster County\tH1\n83226\t16037\tChallis\tID\tCuster County\tH1\n83255\t16037\tMoore\tID\tCuster County\tH1\n83227\t16037\tClayton\tID\tCuster County\tH1\n83278\t16037\tStanley\tID\tCuster County\tH1\n83235\t16037\tEllis\tID\tCuster County\tH1\n83251\t16037\tMackay\tID\tCuster County\tH1\n83648\t16039\tMountain home afb\tID\tElmore County\tH1\n83623\t16039\tGlenns ferry\tID\tElmore County\tH1\n83327\t16039\tFairfield\tID\tElmore County\tH1\n83627\t16039\tHammett\tID\tElmore County\tH1\n83633\t16039\tKing hill\tID\tElmore County\tH1\n83647\t16039\tMountain home\tID\tElmore County\tH1\n83624\t16039\tGrand view\tID\tElmore County\tH1\n83716\t16039\tBoise\tID\tElmore County\tH1\n83237\t16041\tFranklin\tID\tFranklin County\tH1\n83228\t16041\tClifton\tID\tFranklin County\tH1\n83286\t16041\tWeston\tID\tFranklin County\tH1\n83232\t16041\tDayton\tID\tFranklin County\tH1\n83241\t16041\tGrace\tID\tFranklin County\tH1\n83283\t16041\tThatcher\tID\tFranklin County\tH1\n83263\t16041\tPreston\tID\tFranklin County\tH1\n83425\t16043\tHamer\tID\tFremont County\tH1\n83448\t16043\tSugar 
